vi "main_3.vi"(1 "DLL Type":T2, 5 "Input 1":dbl, 7 "Input 2":dbl, 11 "error in (no error)":errorcluster, 12 "Operation":T1) -> (6 "Output":dbl, 15 "error out":errorcluster)   [LabVIEW 2023, in "task_3.lvlib"]
doc: "Used to select the DLL and run the operations."
uses:
  task_3.lvlib
  Controls/dll_selector.ctl
  Controls/operation_selector.ctl
  <vilib>/Utility/error.llb/DialogType.ctl
  D:/labview/TIPS/builds/assignmrnt_11/Math_net/MathNet_lab.dll
  builds/assignmrnt_11/Math_net/MathNet_lab.dll
  builds/assignmrnt_11/Math/MathC_lab.dll
panel:
  in  "Stop":bool
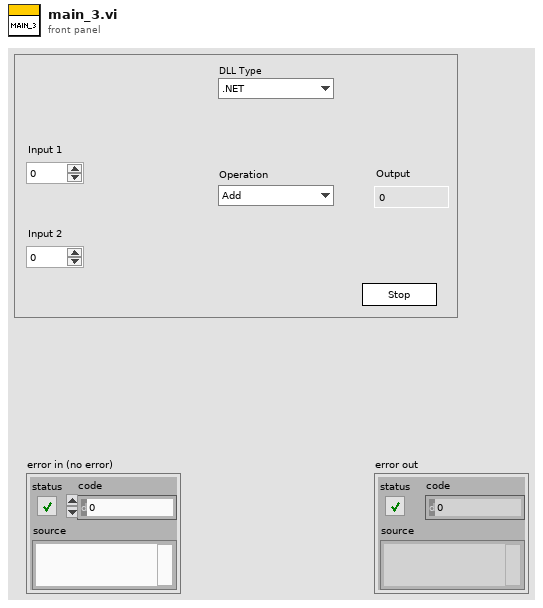
[diagram p1: front panel]
types:
  T1 = typedef "operation_selector.ctl" = enum16{"Add", "Subtract", "Divide", "Multiply"}
  T2 = typedef "dll_selector.ctl" = enum16{".NET", "C DLL"}
  T3 = typedef "DialogType.ctl" = u16
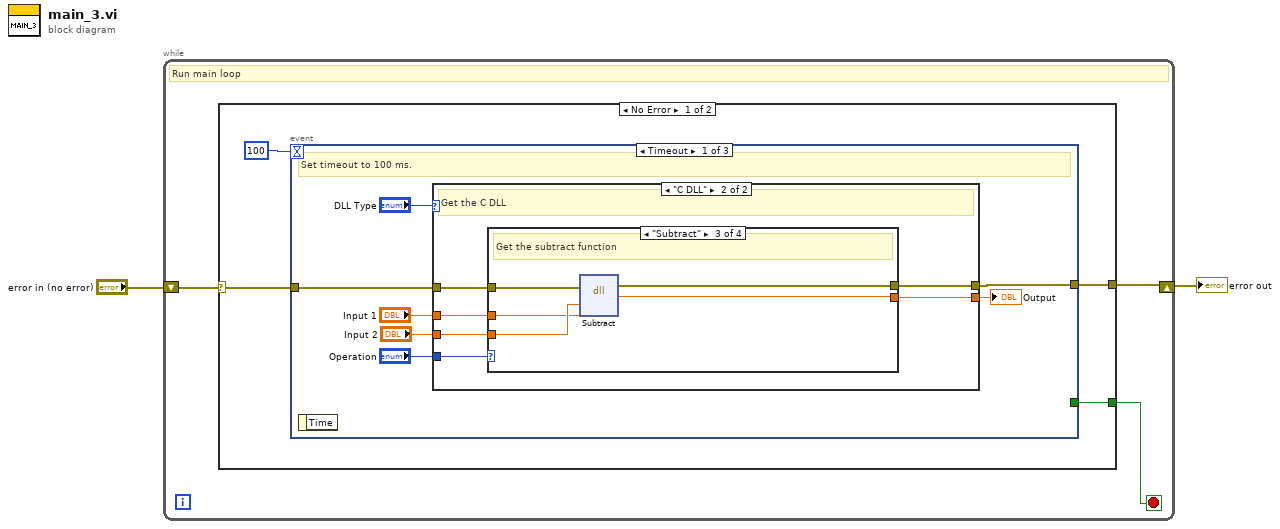
[diagram p0: block diagram]
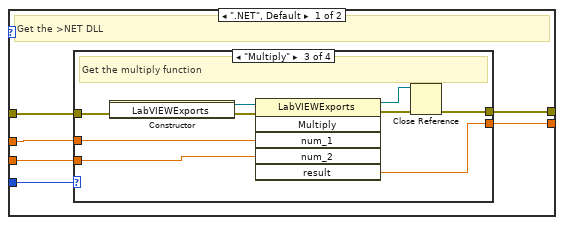
[diagram p2: hidden frame]
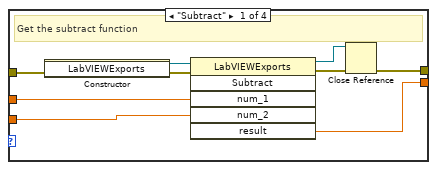
[diagram p3: hidden frame]
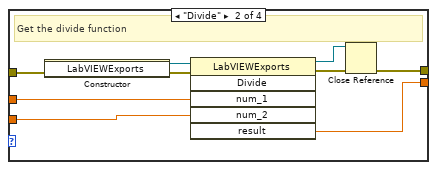
[diagram p4: hidden frame]
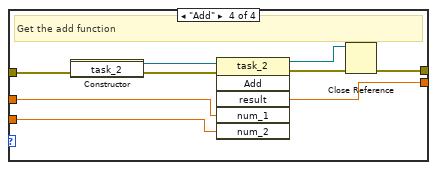
[diagram p5: hidden frame]
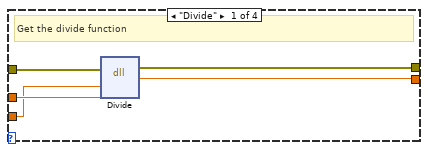
[diagram p6: hidden frame]
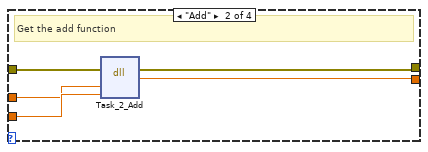
[diagram p7: hidden frame]
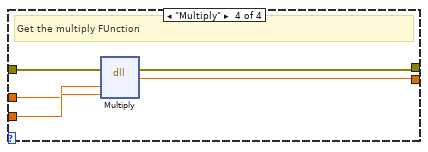
[diagram p8: hidden frame]
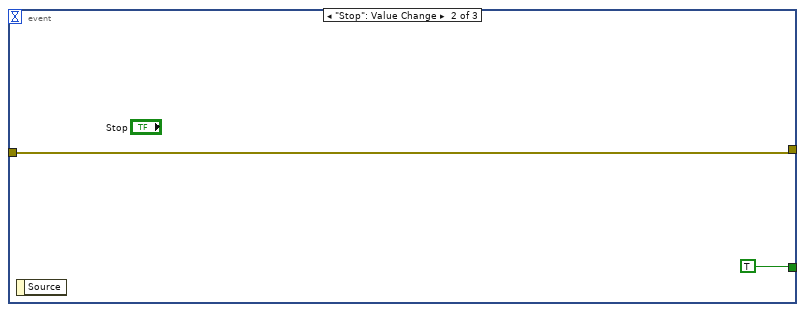
[diagram p9: hidden frame]
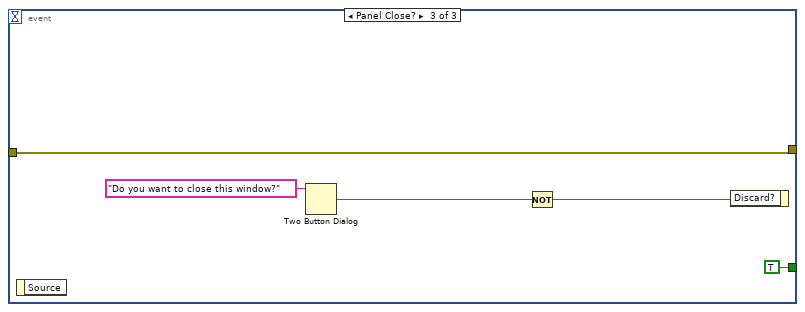
[diagram p10: hidden frame]
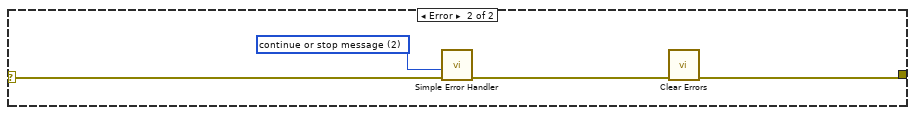
[diagram p11: hidden frame]
diagram:
  n1 = while {
    shift-right: [w4] -> w1
    shift-left: "error in (no error)" -> [w5]
    stop <- w3 stop-if-true
    # "Run main loop"
    n2 = case shown="No Error" w5 {
      selector: w5 -> [w8 w95]
      tunnel: [w7 w92] -> w4
      tunnel: [w6 _] -> w3
      frame No Error {
        n3 = event shown="[0] Timeout" {
          selector: _ -> [_ _ _]
          dyn-events: _ -> [_ _ _]
          timeout: 100 -> [_ _ _]
          tunnel: w8 -> [w11 w85 w91]
          tunnel: [w10 w85 w91] -> w7
          tunnel: [_ TRUE TRUE] -> w6
          event Timeout {
            # "Set timeout to 100 ms."
            n4 = event-data() -> ()  [unwired: 1 in, 1 out]
            n5 = case shown="\"C DLL\"" "DLL Type" {
              tunnel: "Operation" -> [w22 w64]
              tunnel: "Input 1" -> [w20 w60]
              tunnel: "Input 2" -> [w19 w59]
              tunnel: [w18 w63] -> w12
              tunnel: w11 -> [w21 w62]
              tunnel: [w17 w61] -> w10
              frame ".NET", Default {
                # "Get the >NET DLL"
                n6 = case shown="\"Multiply\"" w22 {
                  tunnel: w21 -> [w29 w38 w47 w56]
                  tunnel: w20 -> [w28 w37 w46 w52]
                  tunnel: w19 -> [w27 w36 w45 w51]
                  tunnel: [w26 w35 w44 w50] -> w18
                  tunnel: [w24 w33 w42 w54] -> w17
                  frame "Subtract" {
                    # "Get the subtract function"
                    n7 = constructor class="LabVIEWExports"(error in=w29) -> (reference out=w30:refnum<k24>, error out=w31:errorcluster)  [unwired: 2 in, 1 out]
                    n8 = invoke class="LabVIEWExports" method="Subtract"(reference=w30, error in=w31, "num_1"=w28, "num_2"=w27) -> (reference out=w23:refnum<k24>, error out=w25:errorcluster, "result"=w26:dbl)  [unwired: 2 in, 3 out]
                    n9 = Close Reference(reference=w23, error in (no error)=w25) -> (error out=w24:errorcluster)
                  }
                  frame "Divide" {
                    # "Get the divide function"
                    n10 = constructor class="LabVIEWExports"(error in=w38) -> (reference out=w39:refnum<k24>, error out=w40:errorcluster)  [unwired: 2 in, 1 out]
                    n11 = invoke class="LabVIEWExports" method="Divide"(reference=w39, error in=w40, "num_1"=w37, "num_2"=w36) -> (reference out=w32:refnum<k24>, error out=w34:errorcluster, "result"=w35:dbl)  [unwired: 2 in, 3 out]
                    n12 = Close Reference(reference=w32, error in (no error)=w34) -> (error out=w33:errorcluster)
                  }
                  frame "Multiply" {
                    # "Get the multiply function"
                    n13 = constructor class="LabVIEWExports"(error in=w47) -> (reference out=w48:refnum<k24>, error out=w49:errorcluster)  [unwired: 2 in, 1 out]
                    n14 = invoke class="LabVIEWExports" method="Multiply"(reference=w48, error in=w49, "num_1"=w46, "num_2"=w45) -> (reference out=w41:refnum<k24>, error out=w43:errorcluster, "result"=w44:dbl)  [unwired: 2 in, 3 out]
                    n15 = Close Reference(reference=w41, error in (no error)=w43) -> (error out=w42:errorcluster)
                  }
                  frame "Add" {
                    # "Get the add function"
                    n16 = constructor class="task_2"(error in=w56) -> (reference out=w57:refnum<k24>, error out=w58:errorcluster)  [unwired: 2 in, 1 out]
                    n17 = invoke class="task_2" method="Add"(reference=w57, error in=w58, "num_1"=w52, "num_2"=w51) -> (reference out=w53:refnum<k24>, error out=w55:errorcluster, "result"=w50:dbl)  [unwired: 2 in, 3 out]
                    n18 = Close Reference(reference=w53, error in (no error)=w55) -> (error out=w54:errorcluster)
                  }
                }
              }
              frame "C DLL" {
                # "Get the C DLL"
                n19 = case shown="\"Subtract\"" w64 {
                  tunnel: w60 -> [w66 w73 w75 w83]
                  tunnel: w59 -> [w65 w74 w76 w84]
                  tunnel: [w69 w72 w79 w82] -> w63
                  tunnel: w62 -> [w68 w71 w78 w81]
                  tunnel: [w67 w70 w77 w80] -> w61
                  frame "Divide" {
                    # "Get the divide function"
                    n20 = dll-call lib="D:/labview/TIPS/builds/assignmrnt_11/Math/MathC_lab.dll" fn="Divide"(error in=w68, "num_1"=w65, "num_2"=w66) -> (error out=w67:errorcluster, "return type"=w69:dbl)  [unwired: 4 in, 1 out]
                  }
                  frame "Add" {
                    # "Get the add function"
                    n21 = dll-call lib="D:/labview/TIPS/builds/assignmrnt_11/Math/MathC_lab.dll" fn="Task_2_Add"(error in=w71, "num_1"=w73, "num_2"=w74) -> (error out=w70:errorcluster, "return type"=w72:dbl)  [unwired: 4 in, 1 out]
                  }
                  frame "Subtract" {
                    # "Get the subtract function"
                    n22 = dll-call lib="D:/labview/TIPS/builds/assignmrnt_11/Math/MathC_lab.dll" fn="Subtract"(error in=w78, "num_1"=w76, "num_2"=w75) -> (error out=w77:errorcluster, "return type"=w79:dbl)  [unwired: 4 in, 1 out]
                  }
                  frame "Multiply" {
                    # "Get the multiply FUnction"
                    n23 = dll-call lib="D:/labview/TIPS/builds/assignmrnt_11/Math/MathC_lab.dll" fn="Multiply"(error in=w81, "num_1"=w83, "num_2"=w84) -> (error out=w80:errorcluster, "return type"=w82:dbl)  [unwired: 4 in, 1 out]
                  }
                }
              }
            }
            "Output" <- w12
          }
          event "Stop": Value Change {
            n24 = event-data() -> ()  [unwired: 1 in, 1 out]
          }
          event Panel Close? {
            n25 = event-data() -> ()  [unwired: 1 in, 1 out]
            n26 = Two Button Dialog(message="Do you want to close this window?") -> (T button?=w89:bool)  [unwired: 2 in]
            n27 = Not(x=w89) -> (.not. x?=w88:bool)
            n28 = event-data("Discard?"=w88) -> ()  [unwired: 1 in, 1 out]
          }
        }
      }
      frame Error {
        w93 = T3 2 items=["no dialog", "OK message", "continue or stop message", "OK message + warnings", "continue/stop + warnings"] ("type of dialog (OK msg:1)")
        n29 = call <vilib>:"Simple Error Handler.vi"("type of dialog (OK msg:1)"=w93, "error in (no error)"=w95) -> ("error out"=w94:errorcluster)  [unwired: 3 in, 4 out]
        n30 = call <vilib>:"Clear Errors.vi"("error in (no error)"=w94) -> ("error out"=w92:errorcluster)  [unwired: 5 in, 1 out]
      }
    }
  }
  "error out" <- w1
